vi "Execute-RT-Benchmarking.vi"   [LabVIEW 2014]
uses:
  <vilib>/Utility/error.llb/DialogType.ctl
  <vilib>/Wiresmith Technology/LabVIEW CLI/CLI Class/CLI.lvclass
types:
  T1 = cluster{"time to run VI":u32, "time to start VI":u32, "test_name":string}
  T2 = cluster{"time to run VI":u32, "time to start VI":u32}
  T3 = typedef "DialogType.ctl" = u16
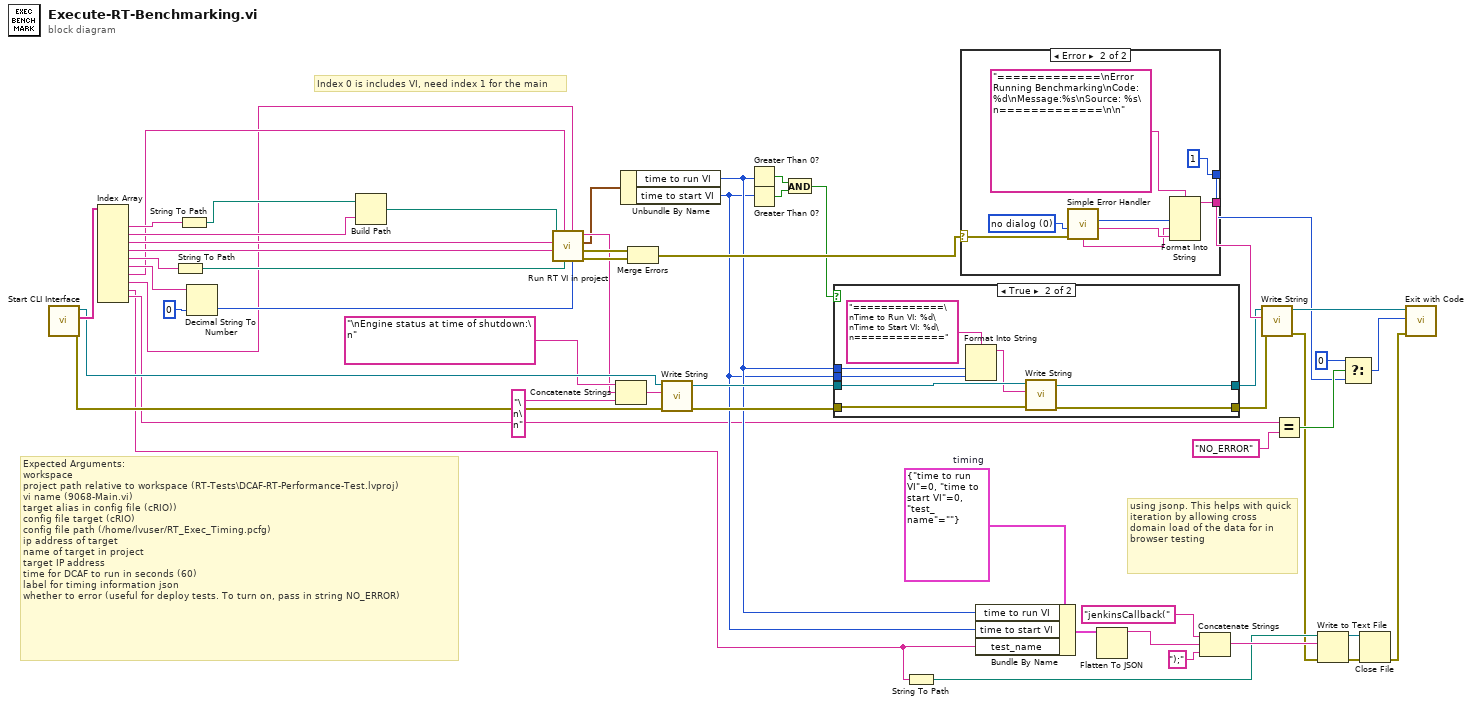
[diagram p0: block diagram]
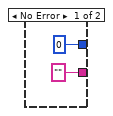
[diagram p3: hidden frame]
diagram:
  w15 = T1 {"time to run VI"=0, "time to start VI"=0, "test_name"=""}  # timing
  # "using jsonp. This helps with quick iteration by allowing cross domain load of the data for in browser testing"
  # "Index 0 is includes VI, need index 1 for the main"
  # "Expected Arguments:\nworkspace \nproject path relative to workspace (RT-Tests\\DCAF-RT-Performance-Test.lvproj)\nvi name (9068-Main.vi)\ntarget alias in config file (cRIO))\nconfig file target (cRIO)\nconfig file path (/home/lvuser/RT_Exec_Timing.pcfg)\nip address of target\nname of target in project\ntarget IP address\ntime for DCAF to run in seconds (60)\nlabel for timing information json\nwhether to error (useful for deploy tests. To turn on, pass in string NO_ERROR)"
  n1 = call <vilib>:"Start CLI Interface.vi"() -> ("error out"=w33:errorcluster, "Custom Parameters"=w53:string[], "CLI out"=w34:refnum<class "CLI.lvclass">)  [unwired: 9 in]
  n2 = Index Array(array=w53) -> (element #1=w37:string, element #2=w46:string, element #3=w44:string, element #4=w43:string, element #5=w48:string, element #6=w49:string, element #7=w36:string, element #8=w29:string, element #9=w1:string, element #10=w2:string)  [unwired: 10 in]
  n3 = String To Path(string=w48) -> (path=w42:path)
  n4 = String To Path(string=w37) -> (path=w47:path)
  n5 = Decimal String To Number(string=w49, default (0L)=u32 0 ("default (0 I32)")) -> (number=w41:u32)  [unwired: 1 in, 1 out]
  n6 = Build Path(base path=w47, name or relative path=w46) -> (appended path=w45:path)
  n7 = call "Run RT VI in project.vi"("Run Time"=w41, "project target"=w29, "configuration file path"=w42, "ip address"=w36, "target alias"=w43, "vi name"=w44, "Project Path"=w45) -> ("error out"=w40:errorcluster, "invoked VI error out"=w39:errorcluster, "timing"=w16:T2, "engine status"=w30:string)  [unwired: 1 in]
  n8 = Concatenate Strings("\nEngine status at time of shutdown:\n" ("string"), w30, "\n\n" ("string")) -> (w35:string)
  n9 = Unbundle By Name(w16) -> ("time to run VI"=w14:u32, "time to start VI"=w13:u32)
  n10 = Merge Errors(w39, w40) -> (w38:errorcluster)
  n11 = call <vilib>:"Write String.vi"("error in (no error)"=w33, "Text to Write"=w35, "CLI in"=w34) -> ("error out"=w18:errorcluster, "CLI out"=w20:refnum<class "CLI.lvclass">)  [unwired: 7 in]
  n12 = Greater Than 0?(x=w14) -> (x > 0?=w22:bool)
  n13 = Greater Than 0?(x=w13) -> (x > 0?=w23:bool)
  n14 = And(x=w22, y=w23) -> (x .and. y?=w21:bool)
  n15 = case shown="True" w21 {
    tunnel: w20 -> [w55 w63]
    tunnel: [w55 w60] -> w19
    tunnel: w18 -> [w54 w62]
    tunnel: [w54 w61] -> w17
    tunnel: w14 -> [_ w58]
    tunnel: w13 -> [_ w57]
    frame False {
    }
    frame True {
      n16 = Format Into String(format string="=============\nTime to Run VI: %d\nTime to Start VI: %d\n=============", w58, w57) -> (resulting string=w59:string)  [unwired: 2 in, 1 out]
      n17 = call <vilib>:"Write String.vi"("error in (no error)"=w62, "Text to Write"=w59, "CLI in"=w63) -> ("error out"=w61:errorcluster, "CLI out"=w60:refnum<class "CLI.lvclass">)  [unwired: 7 in]
    }
  }
  n18 = String To Path(string=w1) -> (path=w5:path)
  n19 = case shown="Error" w38 {
    selector: w38 -> [_ w70]
    tunnel: ["" w66] -> w51
    tunnel: [0 ("Exit Code (0)") 1 ("Exit Code (0)")] -> w26
    frame No Error {
    }
    frame Error {
      w71 = T3 0 items=["no dialog", "OK message", "continue or stop message", "OK message + warnings", "continue/stop + warnings"] ("type of dialog (OK msg:1)")
      n20 = call <vilib>:"Simple Error Handler.vi"("type of dialog (OK msg:1)"=w71, "error in (no error)"=w70) -> ("code out"=w69:i32, "source out"=w68:string, "message"=w67:string)  [unwired: 3 in, 2 out]
      n21 = Format Into String(format string="=============\nError Running Benchmarking\nCode: %d\nMessage:%s\nSource: %s\n=============\n\n", w69, w67, w68) -> (resulting string=w66:string)  [unwired: 2 in, 1 out]
    }
  }
  n22 = Bundle By Name(cluster=w15, "time to run VI"=w14, "time to start VI"=w13, "test_name"=w1) -> (w12:T1)
  n23 = Flatten To JSON(anything=w12) -> (JSON string=w11:string)  [unwired: 2 in, 1 out]
  n24 = Concatenate Strings("jenkinsCallback(" ("string"), w11, ");" ("string")) -> (w8:string)
  n25 = call <vilib>:"Write String.vi"("error in (no error)"=w17, "Text to Write"=w51, "CLI in"=w19) -> ("error out"=w4:errorcluster, "CLI out"=w52:refnum<class "CLI.lvclass">)  [unwired: 7 in]
  n26 = Equal?(x=w2, y="NO_ERROR") -> (x = y?=w27:bool)
  n27 = Write to Text File(file (use dialog)=w5, text=w8, error in=w4) -> (refnum out=w7:refnum<file>, error out=w6:errorcluster)  [unwired: 1 in, 1 out]
  n28 = Select(t=0, s=w27, f=w26) -> (s? t:f=w24:i32)
  n29 = Close File(refnum=w7, error in=w6) -> (error out=w3:errorcluster)  [unwired: 1 out]
  n30 = call <vilib>:"Exit with Code.vi"("error in (no error)"=w3, "Exit Code (0)"=w24, "CLI in"=w52) -> ()  [unwired: 8 in, 1 out]
